vi "tableCleaner.vi"(8 "error in (no error)":errorcluster, 9 "K4b2orK5?":bool, 10 "Table in":refnum<vi>, 11 "reference in":refnum<class "Project Panels.lvclass">) -> (0 "error out":errorcluster, 3 "reference out":refnum<class "Project Panels.lvclass">)   [LabVIEW 2015, in "Project Panels.lvclass"]
uses:
  Project Panels.lvclass
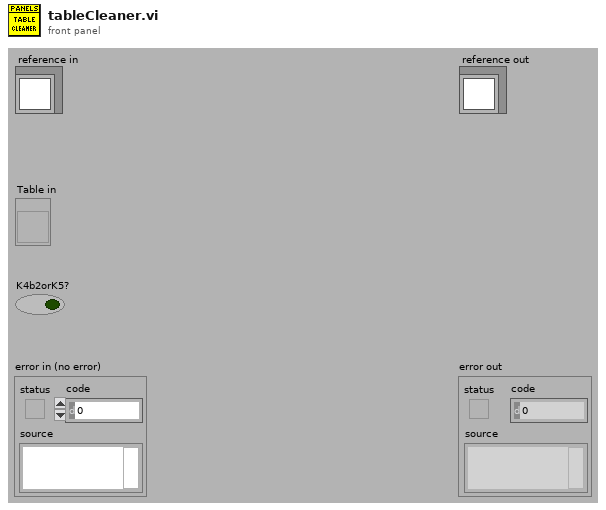
[diagram p1: front panel]
types:
  T1 = enum16{"User-specified Font", "Application Font", "System Font", "Dialog Font"}
  T2 = cluster{"Font Name:":string, "Size":i16, "Strikeout?":bool, "Italic?":bool, "Underline?":bool, "Outline?":bool, "Shadow?":bool, "Bold?":bool}
  T3 = cluster{"left":i16, "top":i16, "right":i16, "bottom":i16}
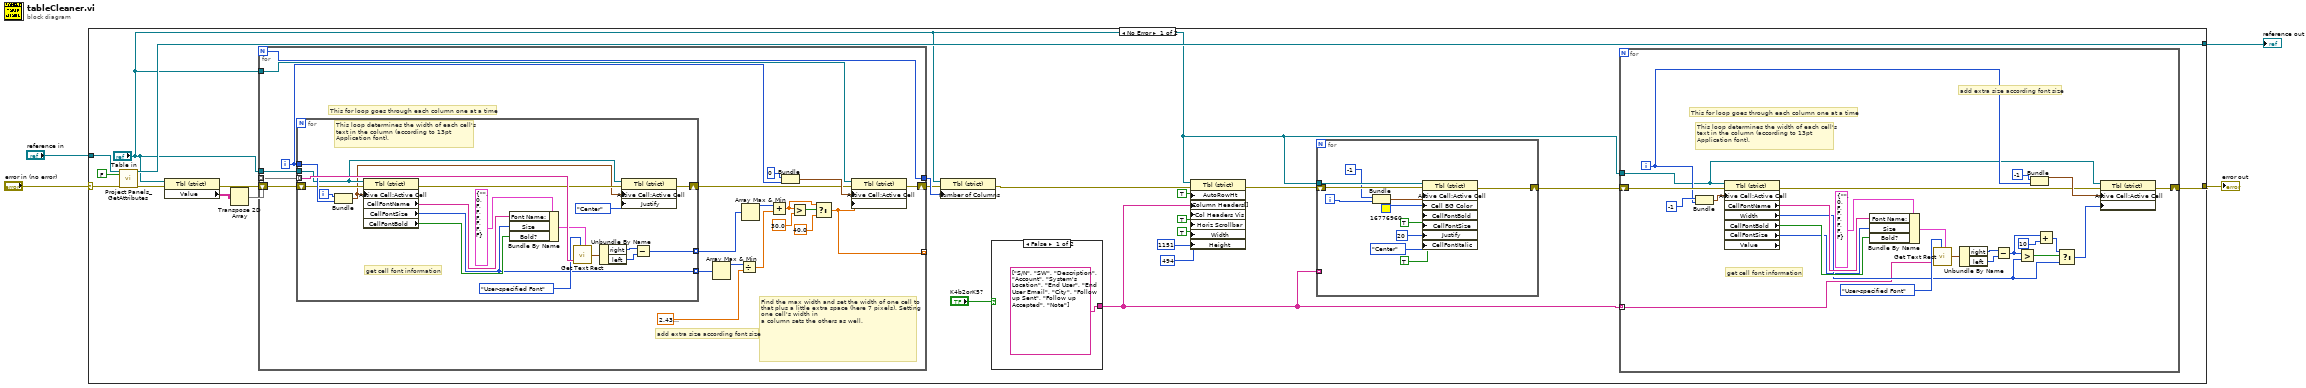
[diagram p0: block diagram]
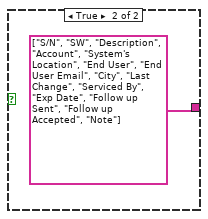
[diagram p2: hidden frame]
diagram:
  n1 = case shown="No Error" "error in (no error)" {
    selector: "error in (no error)" -> [w24 w106]
    tunnel: [w9 w106] -> w3
    tunnel: [w23 w105] -> w1
    tunnel: "reference in" -> [w26 w105]
    frame No Error {
      n2 = call "Project Panels_GetAttributes.vi"("reference in"=w26, "return data? (T)"=FALSE, "error in (no error)"=w24) -> ("reference out"=w23:refnum<class "Project Panels.lvclass">, "error out"=w11:errorcluster)  [unwired: 13 in, 2 out]
      n3 = property on="Property Node" class="Tbl (strict)"(reference="Table in", error in=w11) -> (error out=w18:errorcluster, "Value"=w19:string[][])  [unwired: 1 out]
      n4 = Transpose 2D Array(2D array=w19) -> (transposed array=w20:string[][])
      n5 = for {
        N -> [w74]
        tunnel: w20 -> [w85] mode=indexing
        tunnel: [w74] -> w22
        tunnel: "Table in" -> [w73]
        tunnel: "Table in" -> [w72]
        shift-right: [w75] -> w21
        shift-left: w18 -> [w71]
        tunnel: [w65] -> _ mode=indexing
        i -> [w81]
        # "add extra size according font size"
        # "Find the max width and set the width of one cell to that plus a little extra space (here 7 pixels). Setting one cell's width in\na column sets the others as well."
        # "This for loop goes through each column one at a time"
        n6 = for {
          tunnel: w85 -> [w104] mode=indexing
          tunnel: [w100] -> w84 mode=indexing
          tunnel: w81 -> [w95]
          tunnel: [w92] -> w79 mode=indexing
          tunnel: w73 -> [w87]
          shift-right: [w89] -> w70
          shift-left: w71 -> [w91]
          i -> [w94]
          # "get cell font information"
          # "This loop determines the width of each cell's\ntext in the column (according to 13pt\nApplication font)."
          n7 = Bundle(w94, w95) -> (w86:cluster{i32, i32})  [unwired: 1 in]
          n8 = property on="Property Node" class="Tbl (strict)"(reference=w87, error in=w91, "Active Cell:Active Cell"=w86) -> (error out=w90:errorcluster, "CellFontName"=w99:string, "CellFontSize"=w92:u32, "CellFontBold"=w98:bool)  [unwired: 1 out]
          n9 = Bundle By Name(cluster=T2 {"Font Name:"="", "Size"=0, "Strikeout?"=FALSE, "Italic?"=FALSE, "Underline?"=FALSE, "Outline?"=FALSE, "Shadow?"=FALSE, "Bold?"=FALSE} ("[user-specified font]"), "Font Name:"=w99, "Size"=w92, "Bold?"=w98) -> (w96:T2)
          n10 = call <vilib>:"Get Text Rect.vi"("desired font(Application)"=T1."User-specified Font", "text"=w104, "[user-specified font]"=w96) -> ("rect"=w103:T3)  [unwired: 6 in]
          n11 = Unbundle By Name(w103) -> ("right"=w102:i16, "left"=w101:i16)
          n12 = property on="Property Node" class="Tbl (strict)"(reference=w87, error in=w90, "Active Cell:Active Cell"=w86, "Justify"=enum16{"Left", "Center", "Right"}."Center" ("Active Cell:Cell Justification")) -> (error out=w89:errorcluster)  [unwired: 1 out]
          n13 = Subtract(x=w102, y=w101) -> (x-y=w100:i16)
        }
        n14 = Array Max & Min(array=w79) -> (max value=w78:u32)  [unwired: 3 out]
        n15 = Divide(x=w78, y=sgl 2.43) -> (x/y=w76:sgl)
        n16 = Array Max & Min(array=w84) -> (max value=w80:i16)  [unwired: 3 out]
        n17 = Add(x=w80, y=w76) -> (x+y=w66:sgl)
        n18 = Bundle(0, w81) -> (w82:cluster{i32, i32})  [unwired: 1 in]
        n19 = Greater?(x=w66, y=sgl 30.0) -> (0:w68:bool)
        n20 = Select(t=w66, s=w68, f=sgl 40.0 ("y")) -> (s? t:f=w65:sgl)
        n21 = property on="Property Node" class="Tbl (strict)"(reference=w72, error in=w70, "Active Cell:Active Cell"=w82, "Active Cell:Cell Size:Width"=w65) -> (error out=w75:errorcluster)  [unwired: 1 out]
      }
      n22 = property on="Property Node" class="Tbl (strict)"(reference="Table in", error in=w21, "Number of Columns"=w22) -> (error out=w12:errorcluster)  [unwired: 1 out]
      n23 = case shown="False" "K4b2orK5?" {
        tunnel: [string[] ["S/N", "SW", "Description", "Account", "System's Location", "End User", "End User Email", "City", "Follow up Sent", "Follow up Accepted", "Note"] ("Column Header Strings[]") string[] ["S/N", "SW", "Description", "Account", "System's Location", "End User", "End User Email", "City", "Last Change", "Serviced By", "Exp Date", "Follow up Sent", "Follow up Accepted", "Note"] ("Column Header Strings[]")] -> w5
        frame False {
        }
        frame True {
        }
      }
      n24 = property on="Property Node" class="Tbl (strict)"(reference="Table in", error in=w12, "AutoRowHt"=TRUE ("Autosizing Row Height"), "Column Headers[]"=w5, "Col Headers Vis"=TRUE ("Visible Items:Column Headers Visible"), "Horiz Scrollbar"=TRUE ("Visible Items:Horizontal Scrollbar Visible"), "Width"=u32 1151 ("Size:Width"), "Height"=u32 494 ("Size:Width")) -> (error out=w8:errorcluster)  [unwired: 1 out]
      n25 = for {
        tunnel: "Table in" -> [w35]
        tunnel: w5 -> [_] mode=indexing
        shift-right: [w36] -> w7
        shift-left: w8 -> [w37]
        i -> [w33]
        n26 = Bundle("index"=-1, w33) -> (w34:cluster{"index":i32, i32})  [unwired: 1 in]
        n27 = property on="Property Node" class="Tbl (strict)"(reference=w35, error in=w37, "Active Cell:Active Cell"=w34, "Cell BG Color"=u32 16776960, "CellFontBold"=TRUE ("Active Cell:Cell Font:Bold"), "CellFontSize"=u32 20 ("Active Cell:Cell Font:Size"), "Justify"=enum16{"Left", "Center", "Right"}."Center" ("Active Cell:Cell Justification"), "CellFontItalic"=TRUE ("Active Cell:Cell Font:Italic")) -> (error out=w36:errorcluster)  [unwired: 1 out]
      }
      n28 = for {
        tunnel: "Table in" -> [w41]
        shift-right: [w60] -> w9
        shift-left: w7 -> [w59]
        tunnel: w5 -> [w39] mode=indexing
        i -> [w48]
        # "get cell font information"
        # "This loop determines the width of each cell's\ntext in the column (according to 13pt\nApplication font)."
        # "add extra size according font size"
        # "This for loop goes through each column one at a time"
        n29 = Bundle("index"=-1, w48) -> (w47:cluster{"index":i32, i32})  [unwired: 1 in]
        n30 = property on="Property Node" class="Tbl (strict)" props=["Active Cell:Active Cell", "CellFontName", "Width", "CellFontBold", "CellFontSize", "Value"](reference=w41, error in=w59, "Active Cell:Active Cell"=w47) -> (error out=w38:errorcluster, "CellFontName"=w54:string, "Width"=w42:u32, "CellFontBold"=w53:bool, "CellFontSize"=w40:u32)  [unwired: 2 out]
        n31 = Bundle By Name(cluster=T2 {"Font Name:"="", "Size"=0, "Strikeout?"=FALSE, "Italic?"=FALSE, "Underline?"=FALSE, "Outline?"=FALSE, "Shadow?"=FALSE, "Bold?"=FALSE} ("[user-specified font]"), "Font Name:"=w54, "Size"=w40, "Bold?"=w53) -> (w51:T2)
        n32 = call <vilib>:"Get Text Rect.vi"("desired font(Application)"=T1."User-specified Font", "text"=w39, "[user-specified font]"=w51) -> ("rect"=w57:T3)  [unwired: 6 in]
        n33 = Unbundle By Name(w57) -> ("right"=w56:i16, "left"=w55:i16)
        n34 = Subtract(x=w56, y=w55) -> (x-y=w45:i16)
        n35 = Greater?(x=w45, y=w42) -> (0:w46:bool)
        n36 = Bundle(-1, w48) -> (w61:cluster{i32, i32})  [unwired: 1 in]
        n37 = Add(x=w45, y=i16 10) -> (x+y=w43:i16)
        n38 = Select(t=w43, s=w46, f=w42) -> (s? t:f=w58:u32)
        n39 = property on="Property Node" class="Tbl (strict)"(reference=w41, error in=w38, "Active Cell:Active Cell"=w61, "Active Cell:Cell Size:Width"=w58) -> (error out=w60:errorcluster)  [unwired: 1 out]
      }
    }
    frame Error {
    }
  }
  "error out" <- w3
  "reference out" <- w1
